vi "UNBILITZ-ShutterDriver-Control.vi"(0 "VISA resource name":refnum<visa-resource-name>, 5 "Uniblitz Operation":T3, 7 "Address":T2, 9 "Steady State":T1, 11 "error in (no error)":errorcluster) -> (4 "VISA resource name out":refnum<visa-resource-name>, 15 "error out":errorcluster)   [LabVIEW 2013]
doc: "Provides an interface to all functions for the Uniblitz shutter driver, including:\n\n* Open (refers to opening the shutter)\n* Close (refers to closing the shutter)\n* Trigger\n* Reset\n* AUX Enable\n* AUX Disable\n* Gate On\n* Gate Off"
uses:
  UNIBLITZ-Operation.ctl
  UNIBLITZ-Address.ctl
  UNIBLITZ-SteadyState.ctl
panel:
  # "Inputs"
  # "Outputs"
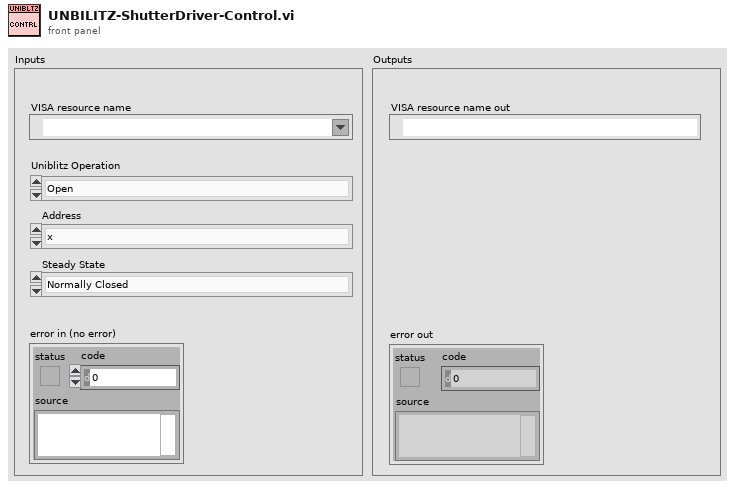
[diagram p1: front panel]
types:
  T1 = typedef "UNIBLITZ-SteadyState.ctl" = enum16{"Normally Closed", "Normally Open"}
  T2 = typedef "UNIBLITZ-Address.ctl" = enum16{"x", "0", "1", "2", "3", "4", "5", "6", "7"}
  T3 = typedef "UNIBLITZ-Operation.ctl" = enum8{"Open", "Close", "Trigger", "Reset", "AUX Enable", "AUX Disable", "Gate On", "Gate Off"}
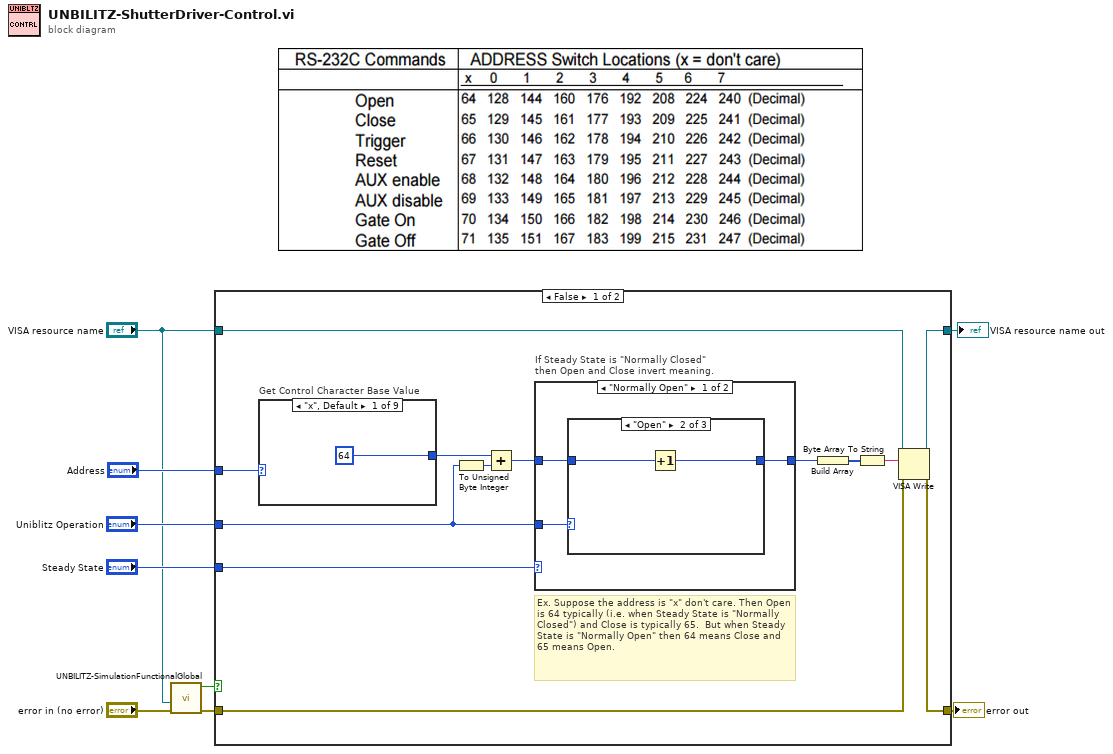
[diagram p0: block diagram]
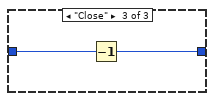
[diagram p3: hidden frame]
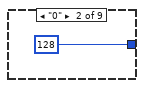
[diagram p5: hidden frame]
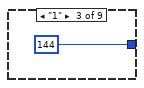
[diagram p6: hidden frame]
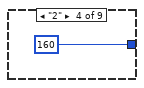
[diagram p7: hidden frame]
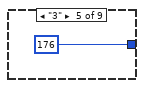
[diagram p8: hidden frame]
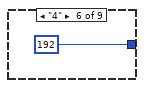
[diagram p9: hidden frame]
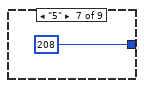
[diagram p10: hidden frame]
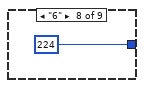
[diagram p11: hidden frame]
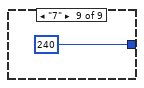
[diagram p12: hidden frame]
diagram:
  n1 = call "UNBILITZ-SimulationFunctionalGlobal.vi"("error in (no error)"="error in (no error)", "VISA Resource Name"="VISA resource name") -> ("error out"=w3:errorcluster, "Simulation Mode"=w2:bool)  [unwired: 8 in]
  n2 = case shown="False" w2 {
    tunnel: "VISA resource name" -> [w22 w42]
    tunnel: [w21 w42] -> w9
    tunnel: [w20 w41] -> w8
    tunnel: "Address" -> [w19 _]
    tunnel: "Steady State" -> [w16 _]
    tunnel: "Uniblitz Operation" -> [w15 _]
    tunnel: w3 -> [w13 w41]
    frame False {
      # "Ex. Suppose the address is \"x\" don't care. Then Open is 64 typically (i.e. when Steady State is \"Normally Closed\") and Close is typically 65.  But when Steady State is \"Normally Open\" then 64 means Close and 65 means Open."
      n3 = case "Get Control Character Base Value" shown="\"x\", Default" w19 {
        tunnel: [u8 64 u8 128 u8 144 u8 160 u8 176 u8 192 u8 208 u8 224 u8 240] -> w18
        frame "x", Default {
        }
        frame "0" {
        }
        frame "1" {
        }
        frame "2" {
        }
        frame "3" {
        }
        frame "4" {
        }
        frame "5" {
        }
        frame "6" {
        }
        frame "7" {
        }
      }
      n4 = To Unsigned Byte Integer(number=w15) -> (unsigned 8bit integer=w17:u8)
      n5 = Add(x=w18, y=w17) -> (x+y=w14:u8)
      n6 = case "If Steady State is \"Normally Closed\" \nthen Open and Close invert meaning." shown="\"Normally Open\"" w16 {
        tunnel: w15 -> [w25 _]
        tunnel: w14 -> [w24 w31]
        tunnel: [w23 w31] -> w11
        frame "Normally Open" {
          n7 = case shown="\"Open\"" w25 {
            tunnel: w24 -> [w26 w28 w30]
            tunnel: [w26 w27 w29] -> w23
            frame Default {
            }
            frame "Open" {
              n8 = Increment(x=w28) -> (x+1=w27:u8)
            }
            frame "Close" {
              n9 = Decrement(x=w30) -> (x-1=w29:u8)
            }
          }
        }
        frame "Normally Closed", Default {
        }
      }
      n10 = Build Array(w11) -> (w12:u8[])
      n11 = Byte Array To String(unsigned byte array=w12) -> (string=w10:string)
      n12 = VISA Write(VISA resource name=w22, write buffer=w10, error in (no error)=w13) -> (VISA resource name out=w21:refnum<visa-resource-name>, error out=w20:errorcluster)  [unwired: 1 out]
    }
    frame True {
    }
  }
  "error out" <- w8
  "VISA resource name out" <- w9
